vi "termometer.vi"() -> ()   [LabVIEW 2017]
panel:
  out "Thermometer Fahrenheit":dbl(slide) scale=0.0..400.0
  in  "Numeric":dbl
  out "Thermometer Celcius":dbl(slide) scale=0.0..100.0
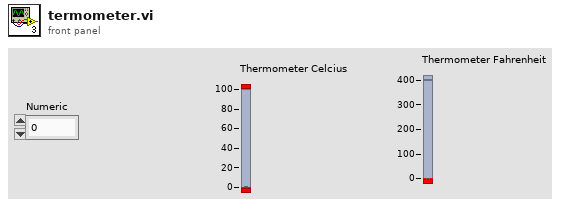
[diagram p1: front panel]
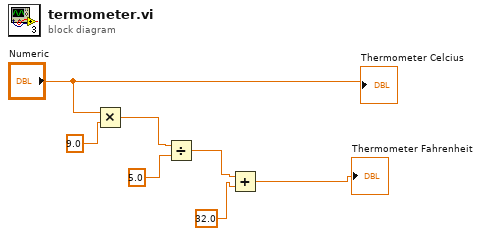
[diagram p0: block diagram]
diagram:
  n1 = Multiply(x="Numeric", y=9.0) -> (x*y=w6:dbl)
  n2 = Divide(x=w6, y=5.0) -> (x/y=w5:dbl)
  n3 = Add(x=w5, y=32.0) -> (x+y=→"Thermometer Fahrenheit":dbl)
  "Thermometer Celcius" <- "Numeric"
